vi "Read Merge in  front.vi"(8 "error in (no error)":errorcluster, 11 "Combined Measurement in":refnum<class "Combined Measurement.lvclass">) -> (0 "error out":errorcluster, 2 "Merge in  front":bool=TRUE, 3 "Combined Measurement out":refnum<class "Combined Measurement.lvclass">)   [LabVIEW 2021, in "Combined Measurement.lvclass"]
uses:
  Combined Measurement.lvclass
  Combined Measurement.lvclass/Combined Measurement.ctl
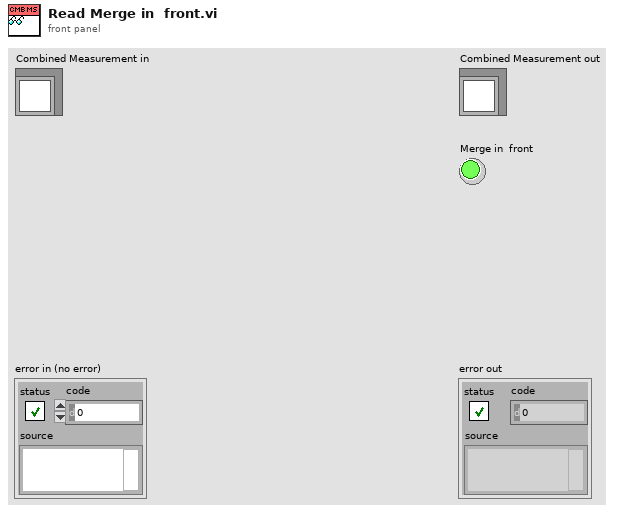
[diagram p1: front panel]
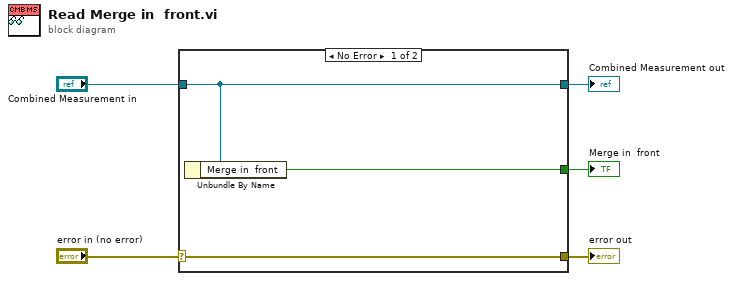
[diagram p0: block diagram]
diagram:
  n1 = case shown="No Error" "error in (no error)" {
    selector: "error in (no error)" -> [w8 w9]
    tunnel: [w8 w9] -> w4
    tunnel: [w7 w10] -> w2
    tunnel: "Combined Measurement in" -> [w7 w10]
    tunnel: [w6 _] -> w1
    frame No Error {
      n2 = Unbundle By Name(w7) -> ("Merge in  front"=w6:bool)
    }
    frame Error {
    }
  }
  "error out" <- w4
  "Combined Measurement out" <- w2
  "Merge in  front" <- w1
